vi "Read Key.vi"(8 "error in (no error)":errorcluster, 11 "[MV] Key Certify in":refnum<class "[MV] Key Certify.lvclass">) -> (0 "error out":errorcluster, 2 "exist?":bool, 3 "[MV] Key Certify out":refnum<class "[MV] Key Certify.lvclass">)   [LabVIEW 2020, in "[MV] Key Certify.lvlib" / "[MV] Key Certify.lvclass"]
uses:
  [MV] Key Certify.lvclass
  <vilib>/registry/registry.llb/Registry RtKey.ctl
  [MV] Key Certify.lvclass/[MV] Key Certify.ctl
  <vilib>/registry/registry.llb/Read Registry Value Simple STR.vi
  <vilib>/YU/YU-Encrypt/Base64/Base64.lvclass
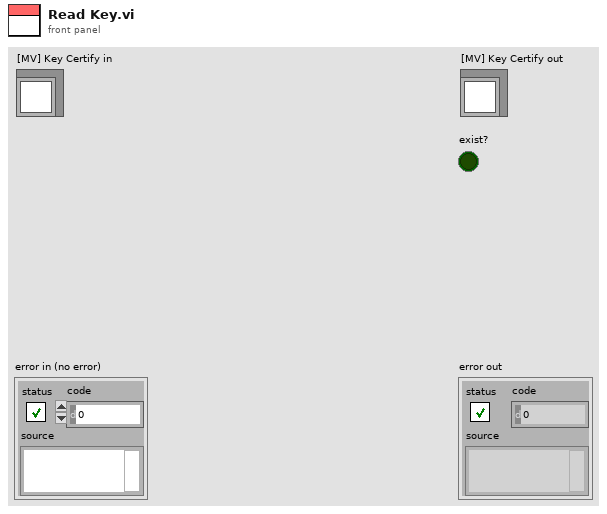
[diagram p1: front panel]
types:
  T1 = typedef "Registry RtKey.ctl" = enum32{"HKEY_CLASSES_ROOT", "HKEY_CURRENT_USER", "HKEY_LOCAL_MACHINE", "HKEY_USERS", "HKEY_PERFORMANCE_DATA", "HKEY_CURRENT_CONFIG", "HKEY_DYN_DATA"}
  T2 = typedef "Registry refnum.ctl" = refnum<k1>
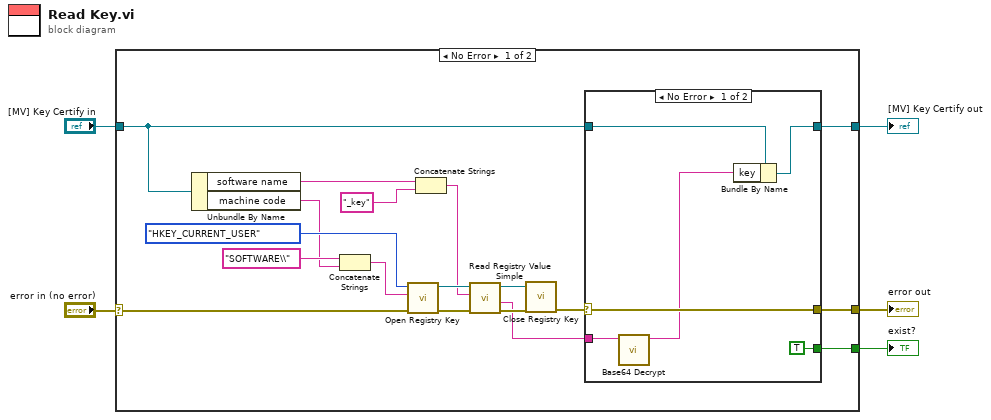
[diagram p0: block diagram]
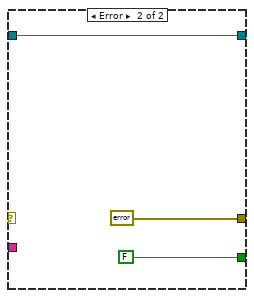
[diagram p2: hidden frame]
diagram:
  n1 = case shown="No Error" "error in (no error)" {
    selector: "error in (no error)" -> [w13 w34]
    tunnel: [w7 w34] -> w4
    tunnel: [w23 w33] -> w2
    tunnel: "[MV] Key Certify in" -> [w12 w33]
    tunnel: [w22 _] -> w1
    frame No Error {
      n2 = Unbundle By Name(w12) -> ("software name"=w10:string, "machine code"=w14:string)
      n3 = Concatenate Strings("SOFTWARE\\" ("subkey"), w14) -> (w16:string)
      n4 = call <vilib>:"Open Registry Key.vi"("error in (no error)"=w13, "subkey"=w16, "root key (HKEY_LOCAL_MACHINE)"=Registry_RtKey."HKEY_CURRENT_USER") -> ("error out"=w21:errorcluster, "refnum out"=w20:T2)  [unwired: 7 in]
      n5 = Concatenate Strings(w10, "_key" ("string")) -> (w9:string)
      n6 = call-poly <vilib>:"Read Registry Value Simple.vi"("error in (no error)"=w21, "value"=w9, "refnum"=w20) -> ("error out"=w18:errorcluster, "String/Binary data"=w6:string, "refnum out"=w19:T2)  [unwired: 3 in, 1 out]
      n7 = call <vilib>:"Close Registry Key.vi"("error in (no error)"=w18, "refnum"=w19) -> ("error out"=w8:errorcluster)  [unwired: 5 in]
      n8 = case shown="No Error" w8 {
        selector: w8 -> [w26 _]
        tunnel: w12 -> [w29 w32]
        tunnel: [w28 w32] -> w23
        tunnel: [TRUE FALSE] -> w22
        tunnel: [w26 errorcluster {"status"=FALSE, "code"=0, "source"=""} ("error IO")] -> w7
        tunnel: w6 -> [w25 _]
        frame No Error {
          n9 = call <vilib>:"Base64 Decrypt.vi"("encrypted data"=w25) -> ("data"=w24:string)  [unwired: 9 in, 1 out]
          n10 = Bundle By Name(cluster=w29, "key"=w24) -> (w28:refnum<class "[MV] Key Certify.lvclass">)
        }
        frame Error {
        }
      }
    }
    frame Error {
    }
  }
  "error out" <- w4
  "[MV] Key Certify out" <- w2
  "exist?" <- w1
